vi "Setup For Triggered Images USB3 v4.3.vi"(5 "error in":errorcluster caption="error in (no error)", 6 "Timeout":u32, 7 "Gain":dbl, 8 "Shutter speed":dbl=0.1, 9 "Camera Name":T3="cam0") -> (0 "Error out":errorcluster caption="error in (no error)", 1 "Session Out":T3="cam0", 2 "Height":u32, 3 "Width":u32, 4 "DeviceID":string)   [LabVIEW 2013]
doc: "The Grab and Attributes Setup VI acquires images continuously and displays the images in an image control using high-level acquisition VIs. The VI also modifes the camera attributes while acquiring images. A grab is appropriate for high-speed applications in which you need to process only one image at a time."
uses:
  <vilib>/userdefined/High Color/IMAQdx.ctl
  <vilib>/vision/driver/IMAQdx.llb/IMAQdx Attribute Type.ctl
  <vilib>/vision/driver/IMAQdx.llb/IMAQdx Attribute Visibility.ctl
  <vilib>/vision/driver/NI_Vision_Acquisition_Software.lvlib
  <resource>/objmgr/imaqdx.rc
panel:
  out "Attribute Information Array":T2(array[cluster])=[{"Attribute Type"=enum."DBL", "Readable"=TRUE, "Writable"=TRUE, "Attribute Name"="CameraAttributes::AnalogControl::Gain"}, {"Attribute Type"=enum."DBL", "Readable"=TRUE, "Writable"=TRUE, "Attribute Name"="CameraAttributes::AnalogControl::BlackLevel"}, {"Attribute Type"=enum."DBL", "Readable"=TRUE, "Writable"=FALSE, "Attribute Name"="CameraAttributes::AnalogControl::Gamma"}, {"Attribute Type"=enum."Bool", "Readable"=TRUE, "Writable"=TRUE, "Attribute Name"="CameraAttributes::AnalogControl::GammaEnabled"}, {"Attribute Type"=enum."I64", "Readable"=TRUE, "Writable"=FALSE, "Attribute Name"="CameraAttributes::AnalogControl::Sharpness"}, {"Attribute Type"=enum."String", "Readable"=TRUE, "Writable"=FALSE, "Attribute Name"="CameraAttributes::DeviceControl::DeviceVendorName"}, {"Attribute Type"=enum."String", "Readable"=TRUE, "Writable"=FALSE, "Attribute Name"="CameraAttributes::DeviceControl::DeviceModelName"}, {"Attribute Type"=enum."String", "Readable"=TRUE, "Writable"=FALSE, "Attribute Name"="CameraAttributes::DeviceControl::DeviceFamilyName"}, {"Attribute Type"=enum."String", "Readable"=TRUE, "Writable"=FALSE, "Attribute Name"="CameraAttributes::DeviceControl::DeviceVersion"}, {"Attribute Type"=enum."String", "Readable"=TRUE, "Writable"=FALSE, "Attribute Name"="CameraAttributes::DeviceControl::DeviceSVNVersion"}, {"Attribute Type"=enum."String", "Readable"=TRUE, "Writable"=FALSE, "Attribute Name"="CameraAttributes::DeviceControl::DeviceID"}, {"Attribute Type"=enum."String", "Readable"=TRUE, "Writable"=TRUE, "Attribute Name"="CameraAttributes::DeviceControl::DeviceUserID"}, {"Attribute Type"=enum."Enum", "Readable"=TRUE, "Writable"=TRUE, "Attribute Name"="CameraAttributes::AcquisitionControl::TriggerSelector"}, {"Attribute Type"=enum."Enum", "Readable"=TRUE, "Writable"=TRUE, "Attribute Name"="CameraAttributes::AcquisitionControl::TriggerMode"}, {"Attribute Type"=enum."Command", "Readable"=FALSE, "Writable"=FALSE, "Attribute Name"="CameraAttributes::AcquisitionControl::TriggerSoftware"}, {"Attribute Type"=enum."Enum", "Readable"=TRUE, "Writable"=TRUE, "Attribute Name"="CameraAttributes::AcquisitionControl::TriggerSource"}, {"Attribute Type"=enum."Enum", "Readable"=TRUE, "Writable"=TRUE, "Attribute Name"="CameraAttributes::AcquisitionControl::TriggerActivation"}, {"Attribute Type"=enum."Enum", "Readable"=TRUE, "Writable"=TRUE, "Attribute Name"="CameraAttributes::AcquisitionControl::ExposureMode"}, {"Attribute Type"=enum."Enum", "Readable"=FALSE, "Writable"=FALSE, "Attribute Name"="CameraAttributes::AcquisitionControl::ExposureAuto"}, {"Attribute Type"=enum."DBL", "Readable"=TRUE, "Writable"=FALSE, "Attribute Name"="CameraAttributes::AcquisitionControl::ExposureTime"}, {"Attribute Type"=enum."Enum", "Readable"=TRUE, "Writable"=TRUE, "Attribute Name"="CameraAttributes::AcquisitionControl::AcquisitionMode"}, {"Attribute Type"=enum."Enum", "Readable"=TRUE, "Writable"=FALSE, "Attribute Name"="CameraAttributes::AcquisitionControl::AcquisitionFrameRateAuto"}, {"Attribute Type"=enum."Bool", "Readable"=FALSE, "Writable"=FALSE, "Attribute Name"="CameraAttributes::AcquisitionControl::AcquisitionFrameRateEnabled"}, {"Attribute Type"=enum."DBL", "Readable"=FALSE, "Writable"=FALSE, "Attribute Name"="CameraAttributes::AcquisitionControl::AcquisitionFrameRate"}, {"Attribute Type"=enum."I64", "Readable"=FALSE, "Writable"=FALSE, "Attribute Name"="CameraAttributes::AcquisitionControl::AcquisitionFrameCount"}, {"Attribute Type"=enum."Enum", "Readable"=TRUE, "Writable"=TRUE, "Attribute Name"="CameraAttributes::ImageFormatControl::PixelFormat"}, {"Attribute Type"=enum."I64", "Readable"=TRUE, "Writable"=TRUE, "Attribute Name"="CameraAttributes::ImageFormatControl::Width"}, {"Attribute Type"=enum."I64", "Readable"=TRUE, "Writable"=TRUE, "Attribute Name"="CameraAttributes::ImageFormatControl::Height"}, {"Attribute Type"=enum."I64", "Readable"=TRUE, "Writable"=TRUE, "Attribute Name"="CameraAttributes::ImageFormatControl::OffsetX"}, {"Attribute Type"=enum."I64", "Readable"=TRUE, "Writable"=TRUE, "Attribute Name"="CameraAttributes::ImageFormatControl::OffsetY"}, {"Attribute Type"=enum."Enum", "Readable"=TRUE, "Writable"=FALSE, "Attribute Name"="CameraAttributes::ImageFormatControl::PixelCoding"}, {"Attribute Type"=enum."I64", "Readable"=TRUE, "Writable"=FALSE, "Attribute Name"="CameraAttributes::ImageFormatControl::PixelDynamicRangeMin"}, {"Attribute Type"=enum."I64", "Readable"=TRUE, "Writable"=FALSE, "Attribute Name"="CameraAttributes::ImageFormatControl::PixelDynamicRangeMax"}, {"Attribute Type"=enum."Enum", "Readable"=TRUE, "Writable"=TRUE, "Attribute Name"="CameraAttributes::ImageFormatControl::TestImageSelector"}, {"Attribute Type"=enum."I64", "Readable"=TRUE, "Writable"=FALSE, "Attribute Name"="CameraAttributes::UserSetControl::UserSetCurrent"}, {"Attribute Type"=enum."Enum", "Readable"=TRUE, "Writable"=TRUE, "Attribute Name"="CameraAttributes::UserSetControl::UserSetSelector"}, {"Attribute Type"=enum."Command", "Readable"=FALSE, "Writable"=TRUE, "Attribute Name"="CameraAttributes::UserSetControl::UserSetLoad"}, {"Attribute Type"=enum."Command", "Readable"=FALSE, "Writable"=TRUE, "Attribute Name"="CameraAttributes::UserSetControl::UserSetSave"}, {"Attribute Type"=enum."DBL", "Readable"=FALSE, "Writable"=FALSE, "Attribute Name"="CameraAttributes::DigitalIOControl::StrobeDelay"}, {"Attribute Type"=enum."DBL", "Readable"=FALSE, "Writable"=FALSE, "Attribute Name"="CameraAttributes::DigitalIOControl::StrobeDuration"}]
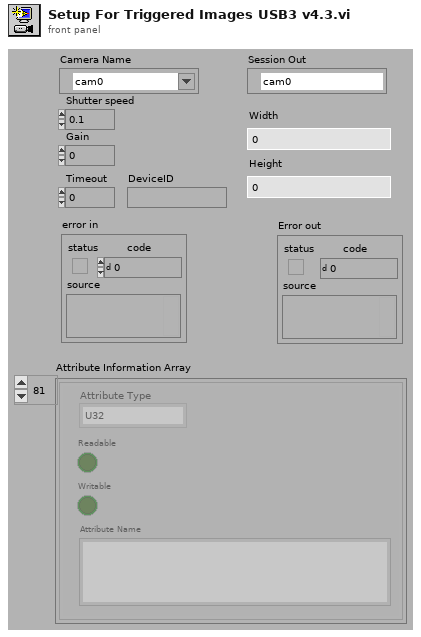
[diagram p1: front panel]
types:
  T1 = typedef "NI_Vision_Acquisition_Software.lvlib/IMAQdx Attribute Type.ctl" = enum32{"U32", "I64", "DBL", "String", "Enum", "Bool", "Command"}
  T2 = cluster{"Attribute Type":T1, "Readable":bool, "Writable":bool, "Attribute Name":string}[]
  T3 = typedef "IMAQdx.ctl" = refnum<k21>
  T4 = typedef "NI_Vision_Acquisition_Software.lvlib/IMAQdx Attribute Visibility.ctl" = enum32{"Simple", "Intermediate", "Advanced"}
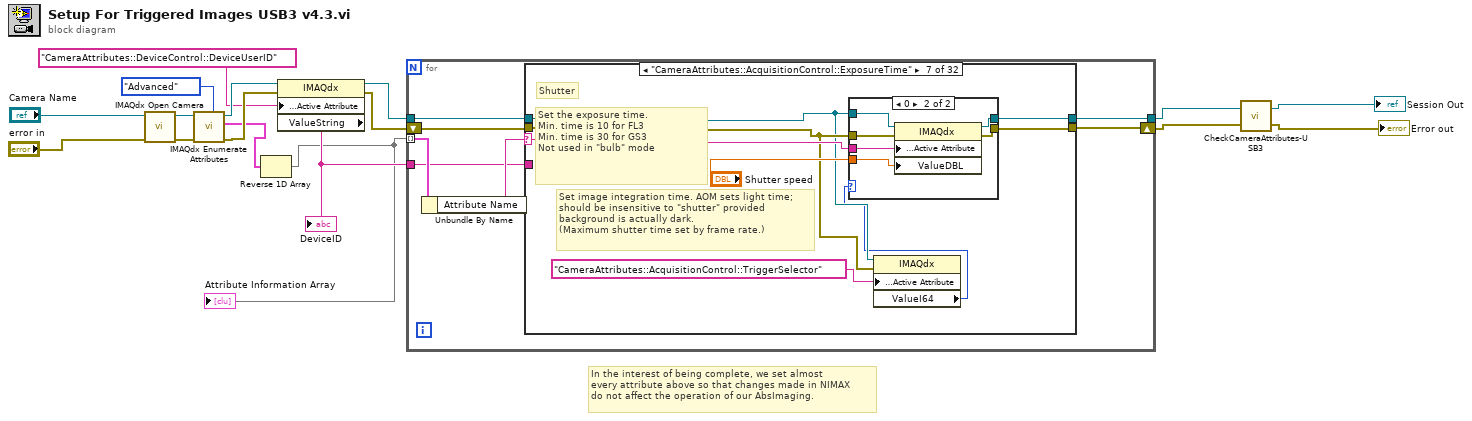
[diagram p0: block diagram]
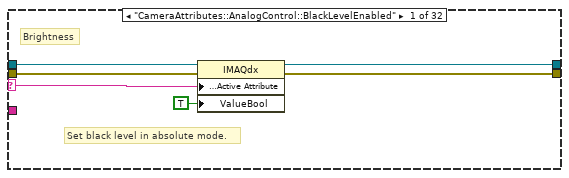
[diagram p2: hidden frame]
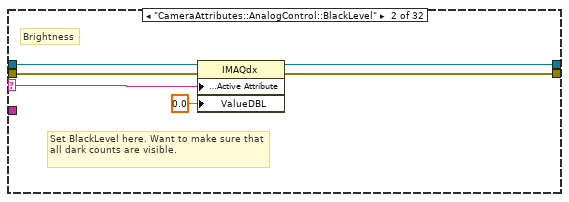
[diagram p3: hidden frame]
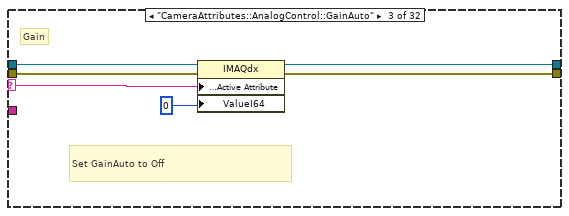
[diagram p4: hidden frame]
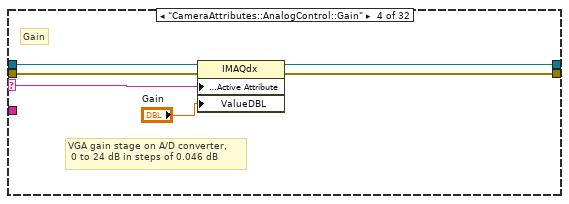
[diagram p5: hidden frame]
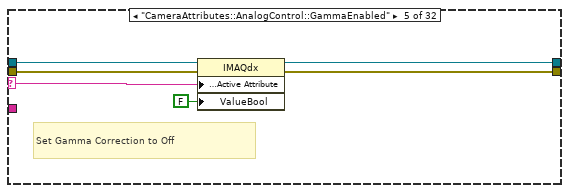
[diagram p6: hidden frame]
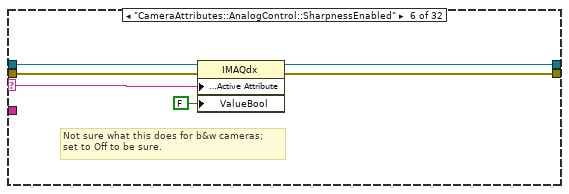
[diagram p7: hidden frame]
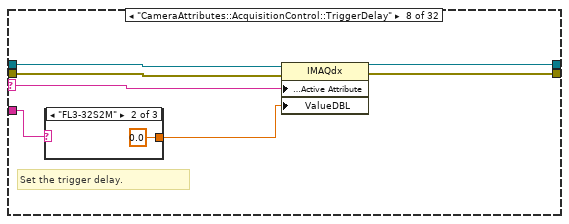
[diagram p9: hidden frame]
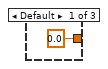
[diagram p10: hidden frame]
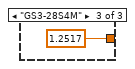
[diagram p11: hidden frame]
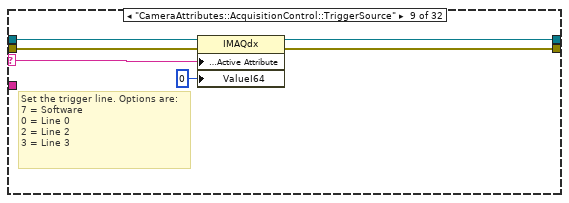
[diagram p12: hidden frame]
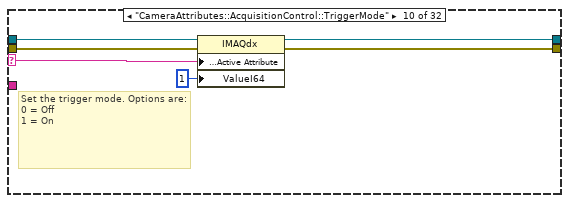
[diagram p13: hidden frame]
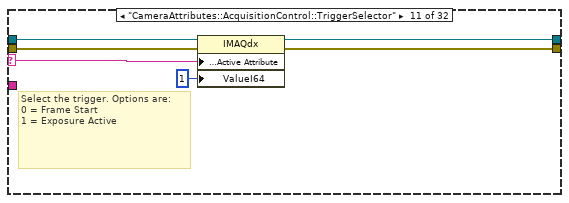
[diagram p14: hidden frame]
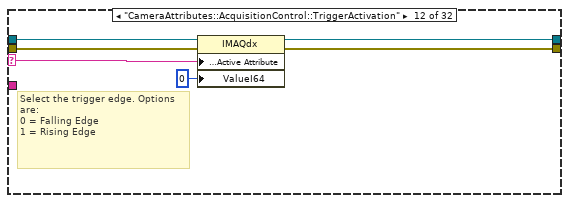
[diagram p15: hidden frame]
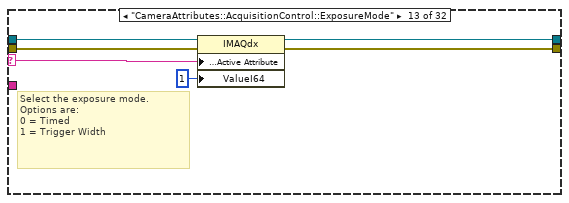
[diagram p16: hidden frame]
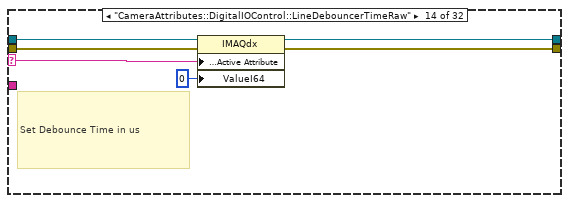
[diagram p17: hidden frame]
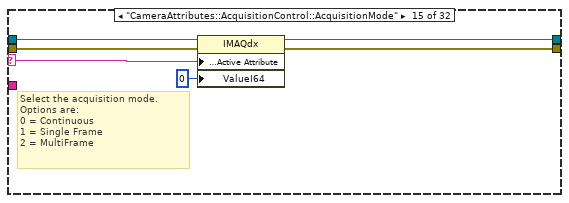
[diagram p18: hidden frame]
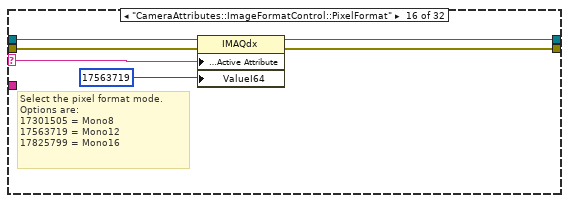
[diagram p19: hidden frame]
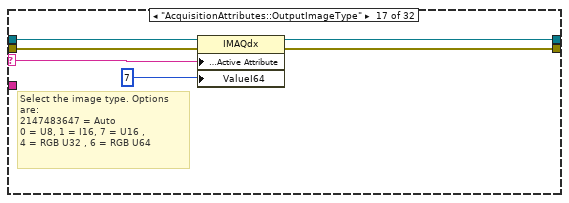
[diagram p20: hidden frame]
diagram:
  # "In the interest of being complete, we set almost\nevery attribute above so that changes made in NIMAX\ndo not affect the operation of our AbsImaging."
  n1 = call <vilib>:"IMAQdx Open Camera.vi"("error in"="error in", "Session In"="Camera Name") -> ("error out"=w15:errorcluster, "Session Out"=w16:T3)  [unwired: 1 in, 7 out]
  n2 = call <vilib>:"IMAQdx Enumerate Attributes.vi"("Visibility"=IMAQdx_Attribute_Visibility."Advanced", "error in"=w15, "Session In"=w16) -> ("error out"=w11:errorcluster, "Attribute Information Array"=w2:T2, "Session Out"=w12:T3)  [unwired: 1 in, 5 out]
  n3 = Reverse 1D Array(array=w2) -> (reversed array=w1:T2)
  "Attribute Information Array" <- w1
  n4 = property class="IMAQdx"(reference=w12, error in=w11, "Camera Attributes:Active Attribute"="CameraAttributes::DeviceControl::DeviceUserID" ("ActiveAttribute")) -> (reference out=w9:T3, error out=w10:errorcluster, "ValueString"=w8:string)
  "DeviceID" <- w8
  n5 = for {
    tunnel: w1 -> [w24] mode=indexing
    tunnel: w9 -> [w19]
    tunnel: [w22] -> w5
    shift-right: [w21] -> w6
    shift-left: w10 -> [w20]
    tunnel: w8 -> [w18]
    n6 = Unbundle By Name(w24) -> ("Attribute Name"=w23:string)
    n7 = case shown="\"CameraAttributes::AcquisitionControl::ExposureTime\"" w23 {
      selector: w23 -> [w26 w32 w38 w44 w50 w56 w67 w79 w88 w94 w100 w106 w112 w118 w124 w130 w136 w142 w148 w154 w162 w172 w181 w187 w193 w199 w205 w210 w216 w222 w228 _]
      tunnel: w19 -> [w30 w36 w42 w48 w54 w60 w62 w83 w92 w98 w104 w110 w116 w122 w128 w134 w140 w146 w152 w158 w161 w171 w180 w186 w192 w198 w204 w214 w220 w226 w232 w234]
      tunnel: w20 -> [w29 w35 w41 w47 w53 w59 w63 w82 w91 w97 w103 w109 w115 w121 w127 w133 w139 w145 w151 w157 w165 w175 w184 w190 w196 w202 w208 w213 w219 w225 w231 w233]
      tunnel: [w28 w34 w40 w46 w52 w58 w66 w81 w90 w96 w102 w108 w114 w120 w126 w132 w138 w144 w150 w156 w164 w174 w183 w189 w195 w201 w207 w212 w218 w224 w230 w234] -> w22
      tunnel: [w27 w33 w39 w45 w51 w57 w65 w80 w89 w95 w101 w107 w113 w119 w125 w131 w137 w143 w149 w155 w163 w173 w182 w188 w194 w200 w206 w211 w217 w223 w229 w233] -> w21
      tunnel: w18 -> [_ _ _ _ _ _ _ w78 _ _ _ _ _ _ _ _ _ _ _ _ w160 w170 _ _ _ _ _ _ _ _ _ _]
      frame "CameraAttributes::AnalogControl::BlackLevelEnabled" {
        # "Set black level in absolute mode."
        # "Brightness"
        n8 = property class="IMAQdx"(reference=w30, error in=w29, "Camera Attributes:Active Attribute"=w26, "ValueBool"=TRUE) -> (reference out=w28:T3, error out=w27:errorcluster)
      }
      frame "CameraAttributes::AnalogControl::BlackLevel" {
        # "Set BlackLevel here. Want to make sure that all dark counts are visible."
        # "Brightness"
        n9 = property class="IMAQdx"(reference=w36, error in=w35, "Camera Attributes:Active Attribute"=w32, "ValueDBL"=0.0) -> (reference out=w34:T3, error out=w33:errorcluster)
      }
      frame "CameraAttributes::AnalogControl::GainAuto" {
        # "Set GainAuto to Off"
        # "Gain"
        n10 = property class="IMAQdx"(reference=w42, error in=w41, "Camera Attributes:Active Attribute"=w38, "ValueI64"=i64 0) -> (reference out=w40:T3, error out=w39:errorcluster)
      }
      frame "CameraAttributes::AnalogControl::Gain" {
        # "VGA gain stage on A/D converter,\n 0 to 24 dB in steps of 0.046 dB"
        # "Gain"
        n11 = property class="IMAQdx"(reference=w48, error in=w47, "Camera Attributes:Active Attribute"=w44, "ValueDBL"="Gain") -> (reference out=w46:T3, error out=w45:errorcluster)
      }
      frame "CameraAttributes::AnalogControl::GammaEnabled" {
        # "Set Gamma Correction to Off"
        n12 = property class="IMAQdx"(reference=w54, error in=w53, "Camera Attributes:Active Attribute"=w50, "ValueBool"=FALSE) -> (reference out=w52:T3, error out=w51:errorcluster)
      }
      frame "CameraAttributes::AnalogControl::SharpnessEnabled" {
        # "Not sure what this does for b&w cameras;\nset to Off to be sure."
        n13 = property class="IMAQdx"(reference=w60, error in=w59, "Camera Attributes:Active Attribute"=w56, "ValueBool"=FALSE) -> (reference out=w58:T3, error out=w57:errorcluster)
      }
      frame "CameraAttributes::AcquisitionControl::ExposureTime" {
        # "Set the exposure time.\nMin. time is 10 for FL3\nMin. time is 30 for GS3\nNot used in \"bulb\" mode"
        # "Set image integration time. AOM sets light time;\nshould be insensitive to \"shutter\" provided \nbackground is actually dark.\n(Maximum shutter time set by frame rate.)"
        # "Shutter"
        n14 = property class="IMAQdx"(reference=w62, error in=w63, "Camera Attributes:Active Attribute"="CameraAttributes::AcquisitionControl::TriggerSelector" ("ActiveAttribute")) -> ("ValueI64"=w61:i64)  [unwired: 2 out]
        n15 = case shown="0" w61 {
          tunnel: "Shutter speed" -> [_ w76]
          tunnel: w67 -> [_ w75]
          tunnel: w63 -> [w69 w74]
          tunnel: w62 -> [w70 w73]
          tunnel: [w70 w72] -> w66
          tunnel: [w69 w71] -> w65
          frame 1, Default {
          }
          frame 0 {
            n16 = property class="IMAQdx"(reference=w73, error in=w74, "Camera Attributes:Active Attribute"=w75, "ValueDBL"=w76) -> (reference out=w72:T3, error out=w71:errorcluster)
          }
        }
      }
      frame "CameraAttributes::AcquisitionControl::TriggerDelay" {
        # "Set the trigger delay."
        n17 = case shown="\"FL3-32S2M\"" w78 {
          tunnel: [0.0 ("ValueDBL") 0.0 ("ValueDBL") 1.2517 ("ValueDBL")] -> w77
          frame Default {
          }
          frame "FL3-32S2M" {
          }
          frame "GS3-28S4M" {
          }
        }
        n18 = property class="IMAQdx"(reference=w83, error in=w82, "Camera Attributes:Active Attribute"=w79, "ValueDBL"=w77) -> (reference out=w81:T3, error out=w80:errorcluster)
      }
      frame "CameraAttributes::AcquisitionControl::TriggerSource" {
        # "Set the trigger line. Options are:\n7 = Software\n0 = Line 0\n2 = Line 2\n3 = Line 3"
        n19 = property class="IMAQdx"(reference=w92, error in=w91, "Camera Attributes:Active Attribute"=w88, "ValueI64"=i64 0) -> (reference out=w90:T3, error out=w89:errorcluster)
      }
      frame "CameraAttributes::AcquisitionControl::TriggerMode" {
        # "Set the trigger mode. Options are:\n0 = Off\n1 = On"
        n20 = property class="IMAQdx"(reference=w98, error in=w97, "Camera Attributes:Active Attribute"=w94, "ValueI64"=i64 1) -> (reference out=w96:T3, error out=w95:errorcluster)
      }
      frame "CameraAttributes::AcquisitionControl::TriggerSelector" {
        # "Select the trigger. Options are:\n0 = Frame Start\n1 = Exposure Active"
        n21 = property class="IMAQdx"(reference=w104, error in=w103, "Camera Attributes:Active Attribute"=w100, "ValueI64"=i64 1) -> (reference out=w102:T3, error out=w101:errorcluster)
      }
      frame "CameraAttributes::AcquisitionControl::TriggerActivation" {
        # "Select the trigger edge. Options are:\n0 = Falling Edge\n1 = Rising Edge"
        n22 = property class="IMAQdx"(reference=w110, error in=w109, "Camera Attributes:Active Attribute"=w106, "ValueI64"=i64 0) -> (reference out=w108:T3, error out=w107:errorcluster)
      }
      frame "CameraAttributes::AcquisitionControl::ExposureMode" {
        # "Select the exposure mode. Options are:\n0 = Timed\n1 = Trigger Width"
        n23 = property class="IMAQdx"(reference=w116, error in=w115, "Camera Attributes:Active Attribute"=w112, "ValueI64"=i64 1) -> (reference out=w114:T3, error out=w113:errorcluster)
      }
      frame "CameraAttributes::DigitalIOControl::LineDebouncerTimeRaw" {
        # "Set Debounce Time in us"
        n24 = property class="IMAQdx"(reference=w122, error in=w121, "Camera Attributes:Active Attribute"=w118, "ValueI64"=i64 0) -> (reference out=w120:T3, error out=w119:errorcluster)
      }
      frame "CameraAttributes::AcquisitionControl::AcquisitionMode" {
        # "Select the acquisition mode. Options are:\n0 = Continuous\n1 = Single Frame\n2 = MultiFrame"
        n25 = property class="IMAQdx"(reference=w128, error in=w127, "Camera Attributes:Active Attribute"=w124, "ValueI64"=i64 0) -> (reference out=w126:T3, error out=w125:errorcluster)
      }
      frame "CameraAttributes::ImageFormatControl::PixelFormat" {
        # "Select the pixel format mode. Options are:\n17301505 = Mono8\n17563719 = Mono12\n17825799 = Mono16"
        n26 = property class="IMAQdx"(reference=w134, error in=w133, "Camera Attributes:Active Attribute"=w130, "ValueI64"=i64 17563719) -> (reference out=w132:T3, error out=w131:errorcluster)
      }
      frame "AcquisitionAttributes::OutputImageType" {
        # "Select the image type. Options are:\n2147483647 = Auto\n0 = U8, 1 = I16, 7 = U16 , \n4 = RGB U32 , 6 = RGB U64"
        n27 = property class="IMAQdx"(reference=w140, error in=w139, "Camera Attributes:Active Attribute"=w136, "ValueI64"=i64 7) -> (reference out=w138:T3, error out=w137:errorcluster)
      }
      frame "CameraAttributes::ImageFormatControl::VideoMode" {
        # "Select the video mode. Options are:\n0 = mode 0, 1 = mode 1\n7 = mode 7, 8 = mode 8"
        n28 = property class="IMAQdx"(reference=w146, error in=w145, "Camera Attributes:Active Attribute"=w142, "ValueI64"=i64 0) -> (reference out=w144:T3, error out=w143:errorcluster)
      }
      frame "CameraAttributes::AcquisitionControl::pgrExposureCompensationAuto" {
        # "Select the exposure compensation mode. Options are:\n0 = off, 2 = continuous"
        n29 = property class="IMAQdx"(reference=w152, error in=w151, "Camera Attributes:Active Attribute"=w148, "ValueU32"=u32 0) -> (reference out=w150:T3, error out=w149:errorcluster)
      }
      frame "CameraAttributes::AcquisitionControl::pgrExposureCompensation" {
        # "Select the exposure compensation in EV\n\n0.001 gives zero"
        n30 = property class="IMAQdx"(reference=w158, error in=w157, "Camera Attributes:Active Attribute"=w154, "ValueDBL"=0.001) -> (reference out=w156:T3, error out=w155:errorcluster)
      }
      frame "CameraAttributes::ImageFormatControl::Width" {
        # "Select the width. Max is 2080 for FL3\nMax is 1928 for GH3"
        n31 = case shown="\"FL3-32S2M\"" w160 {
          tunnel: [i64 100 ("ValueI64") i64 2080 ("ValueI64") i64 1928 ("ValueI64")] -> w159
          frame Default {
          }
          frame "FL3-32S2M" {
          }
          frame "GS3-28S4M" {
          }
        }
        "Width" <- w159
        n32 = property class="IMAQdx"(reference=w161, error in=w165, "Camera Attributes:Active Attribute"=w162, "ValueI64"=w159) -> (reference out=w164:T3, error out=w163:errorcluster)
      }
      frame "CameraAttributes::ImageFormatControl::Height" {
        # "Select the height. Max is 1552 for FL3\nMax is 1448 for GH3"
        n33 = case shown="\"FL3-32S2M\"" w170 {
          tunnel: [i64 100 ("ValueI64") i64 1552 ("ValueI64") i64 1448 ("ValueI64")] -> w169
          frame Default {
          }
          frame "FL3-32S2M" {
          }
          frame "GS3-28S4M" {
          }
        }
        "Height" <- w169
        n34 = property class="IMAQdx"(reference=w171, error in=w175, "Camera Attributes:Active Attribute"=w172, "ValueI64"=w169) -> (reference out=w174:T3, error out=w173:errorcluster)
      }
      frame "CameraAttributes::ImageFormatControl::OffsetX" {
        # "Select the X offset."
        n35 = property class="IMAQdx"(reference=w180, error in=w184, "Camera Attributes:Active Attribute"=w181, "ValueI64"=i64 0) -> (reference out=w183:T3, error out=w182:errorcluster)
      }
      frame "CameraAttributes::ImageFormatControl::OffsetY" {
        # "Select the Y offset."
        n36 = property class="IMAQdx"(reference=w186, error in=w190, "Camera Attributes:Active Attribute"=w187, "ValueI64"=i64 0) -> (reference out=w189:T3, error out=w188:errorcluster)
      }
      frame "CameraAttributes::ImageFormatControl::BinningVertical" {
        # "No vertical binning"
        n37 = property class="IMAQdx"(reference=w192, error in=w196, "Camera Attributes:Active Attribute"=w193, "ValueI64"=i64 1) -> (reference out=w195:T3, error out=w194:errorcluster)
      }
      frame "AcquisitionAttributes::Timeout" {
        # "Set the timeout"
        n38 = property class="IMAQdx"(reference=w198, error in=w202, "Camera Attributes:Active Attribute"=w199, "ValueU32"="Timeout") -> (reference out=w201:T3, error out=w200:errorcluster)
      }
      frame "CameraAttributes::ImageFormatControl::ReverseX" {
        # "Reverse X or not"
        n39 = property class="IMAQdx"(reference=w204, error in=w208, "Camera Attributes:Active Attribute"=w205, "ValueBool"=FALSE) -> (reference out=w207:T3, error out=w206:errorcluster)
      }
      frame "CameraAttributes::AcquisitionControl::TriggerDelayEnabled" {
        # "Do not want any TriggerDelay"
        n40 = property class="IMAQdx"(reference=w214, error in=w213, "Camera Attributes:Active Attribute"=w210, "ValueBool"=FALSE) -> (reference out=w212:T3, error out=w211:errorcluster)
      }
      frame "AcquisitionAttributes::SwapPixelBytes" {
        # "Don't swap bytes"
        n41 = property class="IMAQdx"(reference=w220, error in=w219, "Camera Attributes:Active Attribute"=w216, "ValueBool"=FALSE) -> (reference out=w218:T3, error out=w217:errorcluster)
      }
      frame "AcquisitionAttributes::ShiftPixelBits" {
        # "Don't shift bits"
        n42 = property class="IMAQdx"(reference=w226, error in=w225, "Camera Attributes:Active Attribute"=w222, "ValueBool"=FALSE) -> (reference out=w224:T3, error out=w223:errorcluster)
      }
      frame "CameraAttributes::ImageFormatControl::PixelDefectControl::pgrDefectPixelCorrectionEnable" {
        # "Turn on defect control"
        n43 = property class="IMAQdx"(reference=w232, error in=w231, "Camera Attributes:Active Attribute"=w228, "ValueBool"=TRUE) -> (reference out=w230:T3, error out=w229:errorcluster)
      }
      frame Default {
      }
    }
  }
  n44 = call "CheckCameraAttributes-USB3.vi"("error in"=w6, "Camera Name"=w5) -> ("error out"=→"Error out":errorcluster, "Session Out"=→"Session Out":T3)
